vi "Init.vi"(8 "error in (no error)":errorcluster, 11 "Analyze Fluence and Energy in":refnum<class "Analyze Fluence and Energy.lvclass">) -> (0 "error out":errorcluster, 3 "Analyze Fluence and Energy out":refnum<class "Analyze Fluence and Energy.lvclass">)   [LabVIEW 2014, in "Analyze.lvlib" / "Analyze Fluence and Energy.lvclass"]
uses:
  Analyze Fluence and Energy.lvclass
  Analyze Energy/Analyze Energy.lvclass
  Analyze Fluence/Analyze Fluence.lvclass
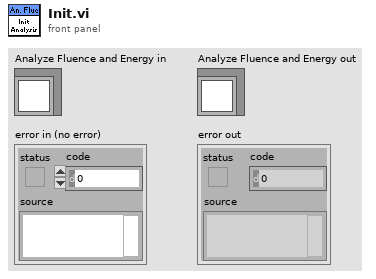
[diagram p1: front panel]
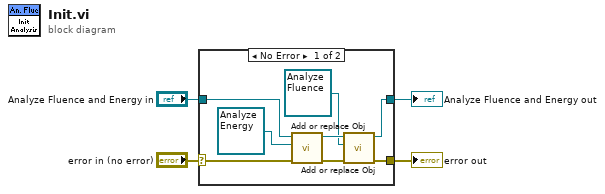
[diagram p0: block diagram]
diagram:
  n1 = case shown="No Error" "error in (no error)" {
    selector: "error in (no error)" -> [w8 w14]
    tunnel: [w7 w14] -> w3
    tunnel: [w9 w13] -> w1
    tunnel: "Analyze Fluence and Energy in" -> [w10 w13]
    frame No Error {
      n2 = call-dynamic "Add or replace Obj.vi"("error in (no error)"=w8, "Analyze Obj"=refnum<class "Analyze Energy.lvclass"> refnum ("Analyze.lvlib:Analyze Energy.lvclass"), "Analyze Compound Analysis Base in"=w10) -> ("error out"=w12:errorcluster, "Analyze Compound Analysis Base out"=w11:refnum<class "Analyze Fluence and Energy.lvclass">)  [unwired: 7 in]
      n3 = call-dynamic "Add or replace Obj.vi"("error in (no error)"=w12, "Analyze Obj"=refnum<class "Analyze Fluence.lvclass"> refnum ("Analyze.lvlib:Analyze Fluence.lvclass"), "Analyze Compound Analysis Base in"=w11) -> ("error out"=w7:errorcluster, "Analyze Compound Analysis Base out"=w9:refnum<class "Analyze Fluence and Energy.lvclass">)  [unwired: 7 in]
    }
    frame Error {
    }
  }
  "error out" <- w3
  "Analyze Fluence and Energy out" <- w1
